vi "simpleArrayWaveformGenerator.vi"(7 "reset signal":bool[](array[boolean]), 8 "error in (no error)":errorcluster, 10 "sampling info":cluster{"Fs":dbl, "#s":dbl}[](array[cluster]), 11 "signal parameters":T1(array[cluster])) -> (0 "error out":errorcluster, 3 "signal(s) in":waveform(dbl)[](array[waveform]))   [LabVIEW 2023]
doc: "Generate simple waveform."
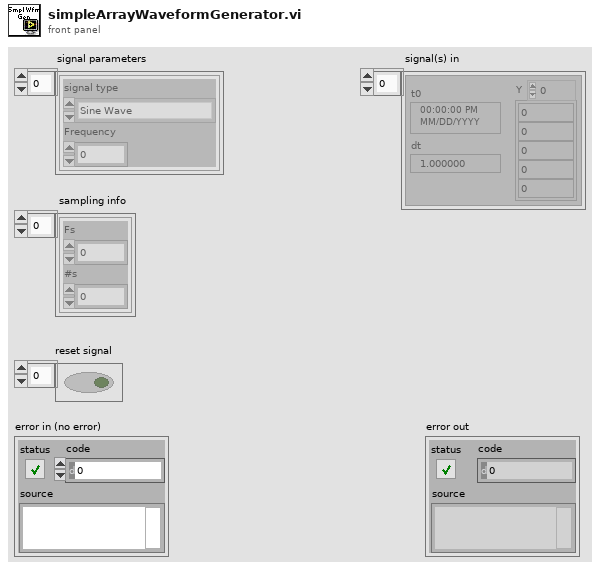
[diagram p1: front panel]
types:
  T1 = cluster{"signal type":enum16{"Sine Wave", "Triangle Wave", "Square Wave", "Sawtooth Wave"}, "Frequency":dbl}[]
  T2 = cluster{"signal type":enum16{"Sine Wave", "Triangle Wave", "Square Wave", "Sawtooth Wave"}, "frequency":dbl, "amplitude":dbl, "phase":dbl, "offset":dbl, "duty cycle (%)":dbl, "reset signal":bool, "sampling info":cluster{"Fs":dbl, "#s":dbl}}
  T3 = enum16{"Sine Wave", "Triangle Wave", "Square Wave", "Sawtooth Wave"}
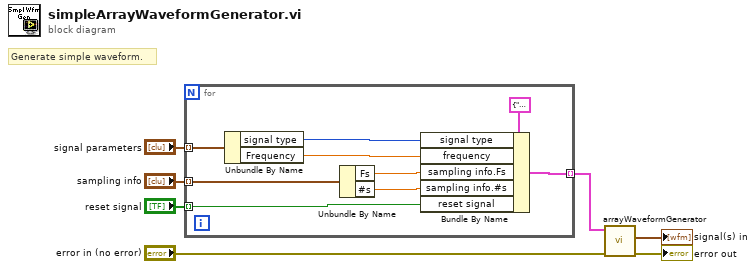
[diagram p0: block diagram]
diagram:
  # "Generate simple waveform."
  n1 = for {
    tunnel: "sampling info" -> [w15] mode=indexing
    tunnel: "signal parameters" -> [w16] mode=indexing
    tunnel: "reset signal" -> [w10] mode=indexing
    tunnel: [w9] -> w6 mode=indexing
    n2 = Unbundle By Name(w16) -> ("signal type"=w14:T3, "Frequency"=w13:dbl)
    n3 = Unbundle By Name(w15) -> ("Fs"=w12:dbl, "#s"=w11:dbl)
    n4 = Bundle By Name(cluster=T2 {"signal type"=enum."Sine Wave", "frequency"=100.0, "amplitude"=1.0, "phase"=0.0, "offset"=0.0, "duty cycle (%)"=50.0, "reset signal"=FALSE, "sampling info"={"Fs"=1000.0, "#s"=1000.0}} ("Signal Generation params"), "signal type"=w14, "frequency"=w13, "sampling info.Fs"=w12, "sampling info.#s"=w11, "reset signal"=w10) -> (w9:T2)
  }
  n5 = call "arrayWaveformGenerator.vi"("error in (no error)"="error in (no error)", "signal generation parameters"=w6) -> ("error out"=→"error out":errorcluster, "signal out"=→"signal(s) in":waveform(dbl)[])  [unwired: 7 in, 1 out]
